vi "Check SSH Connection Status.vi"(8 "Error In":errorcluster, 11 "Install LV Data in":T1={"SSH Session"=refnum, "Status Log"="", "Detailed Log"="", "Credentials"={"Hostname or IP"="192.168.7.2", "Username"="root", "Password"=""}, "Target Info"={"OS Version"="", "CPU"="", "Systemd Version"="", "Internet Access"=FALSE, "Device Type"="", "LV Installed Ver"="", "LV Available Ver"="", "LV Upgrade Available"=FALSE, "Hostname"="", "NIC Info"=[]}, "Reboot Required?"=FALSE}) -> (0 "Error Out":errorcluster, 2 "IsConnected":bool, 3 "Install LV Data":T1={"SSH Session"=refnum, "Status Log"="", "Detailed Log"="", "Credentials"={"Hostname or IP"="192.168.7.2", "Username"="root", "Password"=""}, "Target Info"={"OS Version"="", "CPU"="", "Systemd Version"="", "Internet Access"=FALSE, "Device Type"="", "LV Installed Ver"="", "LV Available Ver"="", "LV Upgrade Available"=FALSE, "Hostname"="", "NIC Info"=[]}, "Reboot Required?"=FALSE})   [LabVIEW 2014, in "LMH-LINX.lvlib"]
uses:
  <vilib>/MakerHub/LINX/LMH-LINX.lvlib
  <vilib>/MakerHub/LINX/Private/Utilties/Target Management/Install LV Data.ctl
  C:/Program Files (x86)/National Instruments/LabVIEW 2014/vi.lib/MakerHub/LINX/Resources/Renci.SshNet.dll
  Resources/Renci.SshNet.dll
  <vilib>/MakerHub/LINX/Private/Utilties/Target Management/Target Info.ctl
  <vilib>/MakerHub/LINX/Private/Utilties/Target Management/NIC Info.ctl
  <vilib>/MakerHub/LINX/Private/Utilties/Target Management/NIC Mode.ctl
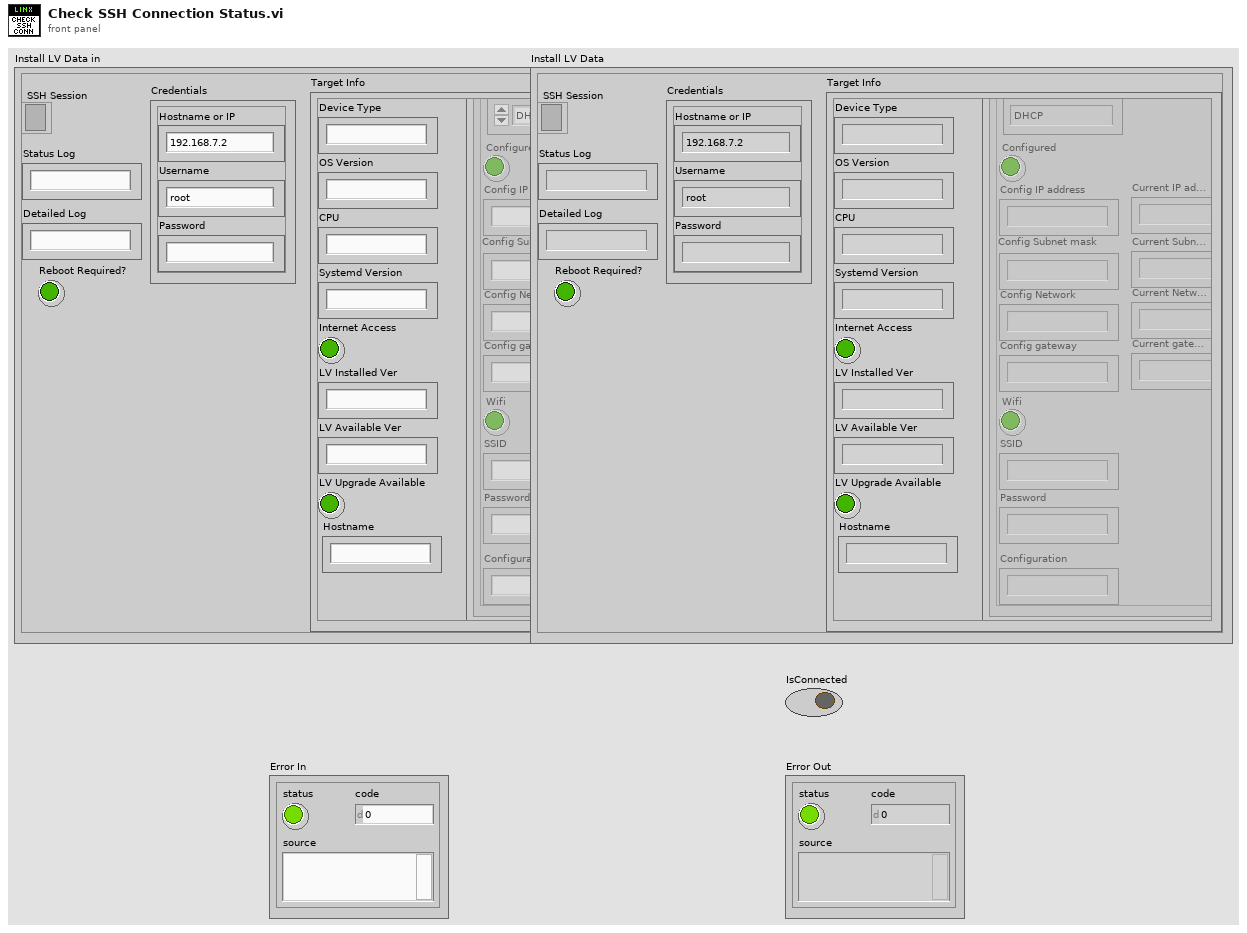
[diagram p1: front panel]
types:
  T1 = typedef "LMH-LINX.lvlib/Install LV Data.ctl" = cluster{"SSH Session":refnum<k24>, "Status Log":string, "Detailed Log":string, "Credentials":cluster{"Hostname or IP":string, "Username":string, "Password":string}, "Target Info":T2, "Reboot Required?":bool}
  T2 = typedef "LMH-LINX.lvlib/Target Info.ctl" = cluster{"OS Version":string, "CPU":string, "Systemd Version":string, "Internet Access":bool, "Device Type":string, "LV Installed Ver":string, "LV Available Ver":string, "LV Upgrade Available":bool, "Hostname":string, "NIC Info":T3[]}
  T3 = typedef "LMH-LINX.lvlib/NIC Info.ctl" = cluster{"Name":string, "NIC Mode":T4, "Configured":bool, "Config IP address":string, "Config Subnet mask":string, "Config Network":string, "Config gateway":string, "Wifi":bool, "SSID":string, "Password":string, "Configuration":string, "Current IP address":string, "Current Subnet mask":string, "Current gateway":string, "Current Network":string}
  T4 = typedef "LMH-LINX.lvlib/NIC Mode.ctl" = enum16{"DHCP", "Static", "Loopback"}
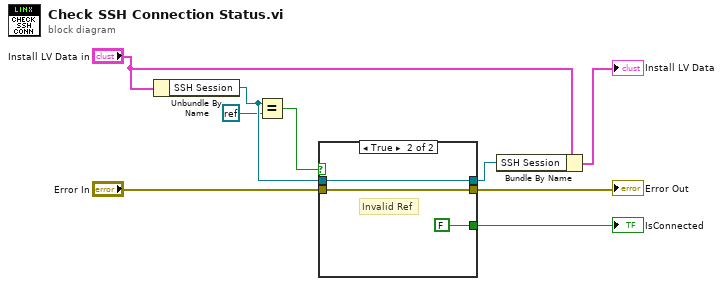
[diagram p0: block diagram]
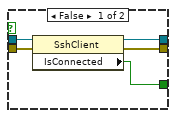
[diagram p2: hidden frame]
diagram:
  n1 = Unbundle By Name("Install LV Data in") -> ("SSH Session"=w6:refnum<k24>)
  n2 = Equal?(x=w6, y=refnum<k0> refnum) -> (x = y?=w5:bool)
  n3 = case shown="True" w5 {
    tunnel: [w12 FALSE] -> w9
    tunnel: w6 -> [w14 w15]
    tunnel: "Error In" -> [w13 w16]
    tunnel: [w11 w15] -> w3
    tunnel: [w10 w16] -> w8
    frame False {
      n4 = property class="SshClient"(reference=w14, error in=w13) -> (reference out=w11:refnum<k24>, error out=w10:errorcluster, "IsConnected"=w12:bool)
    }
    frame True {
      # "Invalid Ref"
    }
  }
  "IsConnected" <- w9
  "Error Out" <- w8
  n5 = Bundle By Name(cluster="Install LV Data in", "SSH Session"=w3) -> (→"Install LV Data":T1)
